vi "Synchronized Linked AI and AO.vi"() -> ()   [LabVIEW 2019, in "GettingStarted_5785_Host.lvlib"]
uses:
  GettingStarted_5785_Host.lvlib
  <vilib>/userDefined/High Color/nirio_resource_hc.ctl
  <instrlib>/FlexRIO/API/Host/v1/NI FlexRIO/API/Reference Clock Source.ctl
  <instrlib>/FlexRIO/API/Host/v1/NI FlexRIO/API/Configure Reference Clock.vi
  <instrlib>/FlexRIO/API/Host/v1/NI FlexRIO/API/Get Property Reference - Fpga Small.vi
  <instrlib>/FlexRIO/API/Host/v1/NI FlexRIO/API/Configure Immediate Start Trigger.vi
  <instrlib>/FlexRIO/API/Host/v1/NI FlexRIO/API/Configure Digital Edge Start Trigger.vi
  <instrlib>/FlexRIO/API/Host/v1/NI FlexRIO/API/Read Stream 1D WDT.vi
  <vilib>/FPGAPlugInAG/Dynamic/niLvFpga_Close_Dynamic.vi
  <vilib>/rvi/interface/nirviCloseFPGA/nirviCloseFPGA.xnode
  <instrlib>/FlexRIO/API/Host/v1/NI FlexRIO API v1.lvlib
  <resource>/objmgr/niflexrioapiStream.rc
  <resource>/objmgr/niflexrioapiTrigger.rc
panel:
  in  "flexrio tranceivers":T2(array[cluster])
  in  "frequency":dbl=32000000.0 format="%0.2p"
  in  "amplitude":dbl=0.2 format="%#_13p"
  in  "sampling info":cluster{"Fs":dbl, "#s":dbl}={"Fs"=3200000000.0, "#s"=1600.0}
  in  "samples to acquire":u64=65536
  out "error out":errorcluster
  out "read data":waveform(dbl)[](graph)=[{"t0"=timestamp(0 s since 1904-01-01), "dt"=3.125e-10, "Y"=[]}, {"t0"=timestamp(0 s since 1904-01-01), "dt"=3.125e-10, "Y"=[]}, {"t0"=timestamp(0 s since 1904-01-01), "dt"=3.125e-10, "Y"=[]}, {"t0"=timestamp(0 s since 1904-01-01), "dt"=3.125e-10, "Y"=[]}]
  out "Output Waveform":waveform(dbl)[](graph)
  in  "trigger source":string(combo)
  in  "trigger mode":enum16{"Immediate", "Digital"}(ring)
  # "This example demonstrates how to synchronize multiple FlexRIO transceivers.\nIn this example, the AO stream is linked to the AI stream, meaning that AO generation will begin after AI acquisition.\n\nFor demonstration, it's suggested to use two transceivers, with AO0 on one device connected to AI0 on the other device.\n\nThe same waveform is downloaded to each each device, and generation will begin on AO0 and AO1 when the start trigger is received. AI0 and AI1 are acquired and plotted when the start trigger is received."
  # "Acquisition trigger configuration"
  # "Digital Trigger configuration"
  # "NOTE: it is expected to see the data zeroed out at the beginning.\nThere are sampling, processing, and propagation delays in the parts, the FPGA\ninterface, etc."
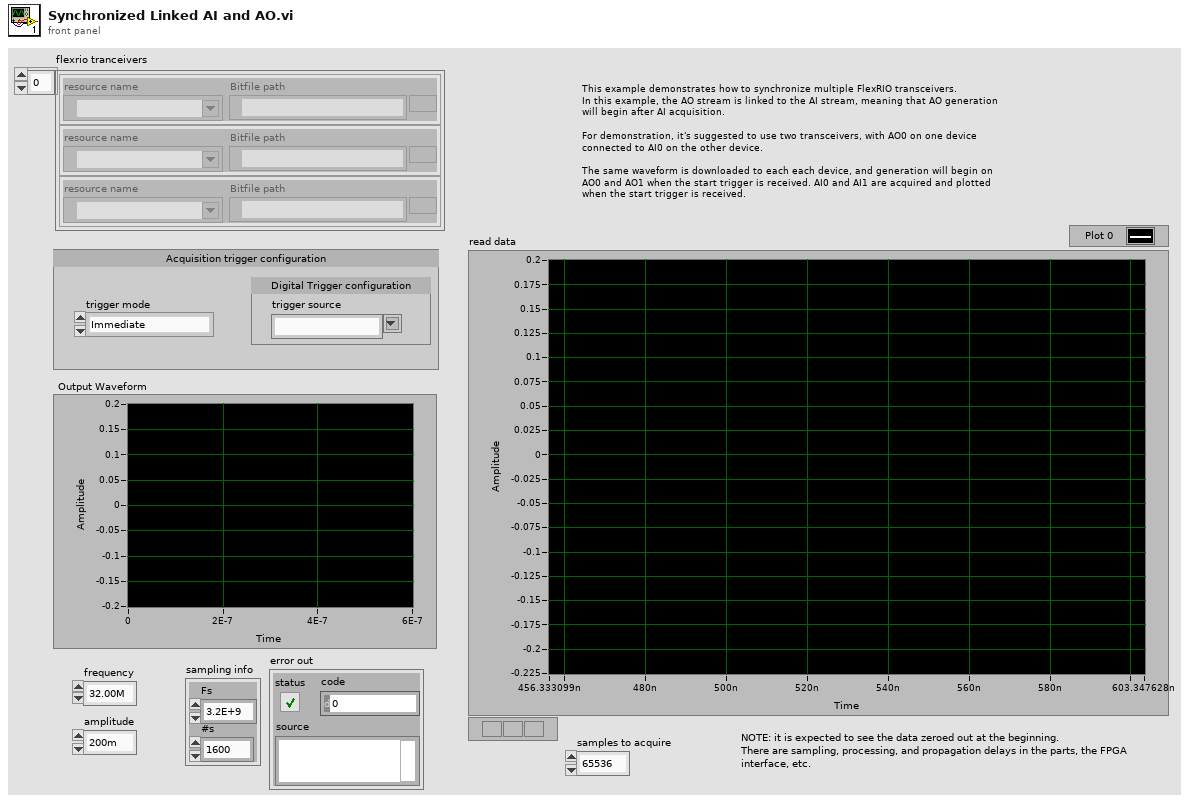
[diagram p1: front panel]
types:
  T1 = typedef "nirio_resource_hc.ctl" = tag
  T2 = cluster{"resource name":T1, "Bitfile path":path}[]
  T3 = typedef "NI FlexRIO API v1.lvlib/Reference Clock Source.ctl" = i32
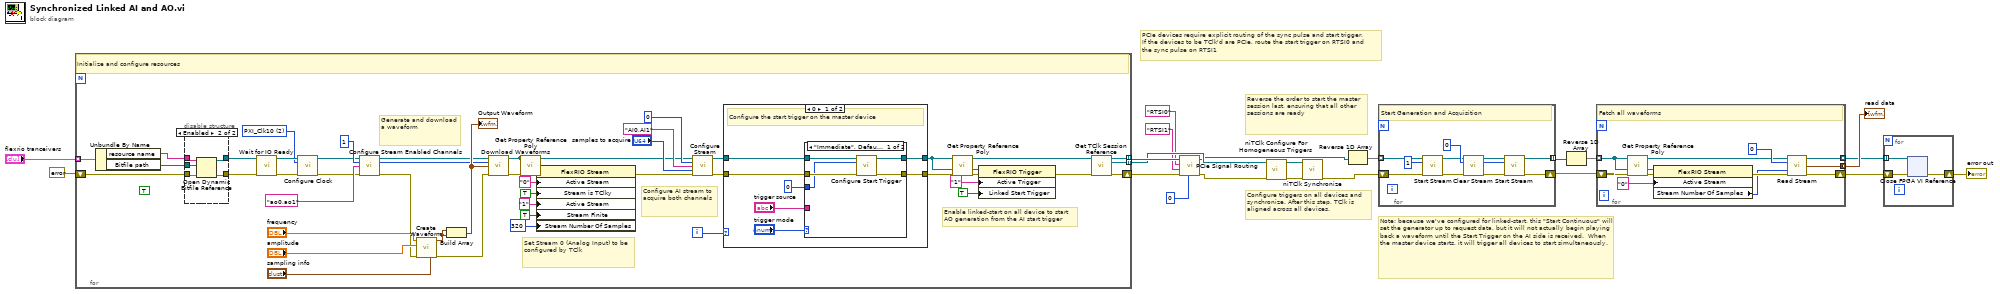
[diagram p0: block diagram]
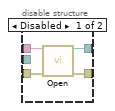
[diagram p2: hidden frame]
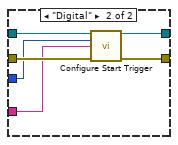
[diagram p3: hidden frame]
diagram:
  # "PCIe devices require explicit routing of the sync pulse and start trigger.\nIf the devices to be TClk'd are PCIe, route the start trigger on RTSI0 and\nthe sync pulse on RTSI1"
  # "Note: because we've configured for linked-start, this \"Start Continuous\" will set the generator up to request data, but it will not actually begin playing back a waveform until the Start Trigger on the AI side is received.  When the master device starts, it will trigger all devices to start simultaneously."
  # "Reverse the order to start the master session last, ensuring that all other sessions are ready"
  # "Configure triggers on all devices and\nsynchronize. After this step, TClk is\naligned across all devices."
  n1 = for {
    shift-right: [w49] -> w7
    shift-left: errorcluster {"status"=FALSE, "code"=0, "source"=""} ("error out") -> [w24]
    tunnel: "flexrio tranceivers" -> [w54] mode=indexing
    tunnel: [w48] -> w8 mode=indexing
    tunnel: [w47] -> w4 mode=indexing
    i -> [w50]
    w30 = T3 2 items=["Default", "Onboard", "PXI_Clk10", "External", "None", "Baseboard Reference"] ("reference clock source")
    (unwired) TRUE ("Run When Loaded")
    # "Enable linked-start on all device to start\nAO generation from the AI start trigger"
    # "Configure AI stream to acquire both channels"
    # "Set Stream 0 (Analog Input) to be configured by TClk"
    # "Generate and download a waveform"
    # "Initialize and configure resources"
    n2 = Unbundle By Name(w54) -> ("resource name"=w23:T1, "Bitfile path"=w22:path)
    n3 = disable-structure shown="Enabled" {
      disable-tunnel: [w73 w77] -> w26
      disable-tunnel: [w72 w78] -> w25
      disable-tunnel: w24 -> [w71 w74]
      disable-tunnel: w23 -> [w70 w76]
      disable-tunnel: w22 -> [_ w75]
      frame Disabled {
        n4 = call <instrlib>:"Open.vi"("RIO Device"=w70, "error in"=w71) -> ("fpga interface out"=w73:refnum<k20>, "error out"=w72:errorcluster)  [unwired: 12 in]
      }
      frame Enabled {
        n5 = Open Dynamic Bitfile Reference(0:w76, 1:w75, 3:w74) -> (5:w77:refnum<k20>, 8:w78:errorcluster)  [unwired: 2 in]
      }
    }
    n6 = call <instrlib>:"Wait for IO Ready.vi"("fpga interface in"=w26, "error in"=w25) -> ("fpga interface out"=w34:refnum<k20>, "error out"=w31:errorcluster)  [unwired: 10 in, 2 out]
    n7 = call-poly <instrlib>:"Configure Clock.vi"("fpga interface in"=w34, "reference clock source"=w30, "error in"=w31) -> ("fpga interface out"=w33:refnum<k20>, "error out"=w32:errorcluster)  [unwired: 11 in]
    n8 = call <instrlib>:"Configure Stream Enabled Channels.vi"("fpga interface in"=w33, "stream instance"=u32 1, "channels enabled"="ao0,ao1", "error in"=w32) -> ("fpga interface out"=w39:refnum<k20>, "stream instance out"=w35:u32, "error out"=w38:errorcluster)  [unwired: 8 in, 1 out]
    n9 = call "Create Waveform.vi"("sampling info"="sampling info", "error in (no error)"=w38, "amplitude"="amplitude", "frequency"="frequency") -> ("error out"=w53:errorcluster, "Output Waveform (V)"=w59:waveform(dbl))  [unwired: 5 in, 1 out]
    n10 = Build Array(w59, w59) -> (w57:waveform(dbl)[])
    "Output Waveform" <- w57
    n11 = call "Download Waveforms.vi"("fpga interface in"=w39, "stream instance"=w35, "waveforms"=w57, "error in"=w53) -> ("fpga interface out"=w58:refnum<k20>, "error out"=w56:errorcluster)  [unwired: 9 in, 1 out]
    n12 = call-poly <instrlib>:"Get Property Reference Poly.vi"("error in (no error)"=w56, "fpga interface in"=w58) -> ("error out"=w69:errorcluster, "property reference"=w68:refnum<k20>)  [unwired: 4 in, 1 out]
    n13 = property class="FlexRIO Stream"(reference=w68, error in=w69, "Active Stream"="0", "Stream is TClky"=TRUE ("Configuration:Stream is TClky"), "Active Stream"="1", "Stream Finite"=TRUE ("Configuration:Finite"), "Stream Number Of Samples"=u64 320) -> (error out=w65:errorcluster)  [unwired: 1 out]
    n14 = call <instrlib>:"Configure Stream.vi"("fpga interface in"=w58, "stream instance"=u32 0, "channels enabled"="AI0,AI1", "num samples"="samples to acquire", "error in"=w65) -> ("fpga interface out"=w52:refnum<k20>, "error out"=w51:errorcluster)  [unwired: 7 in, 2 out]
    n15 = case shown="0" w50 {
      tunnel: [w83 w98] -> w40
      tunnel: w52 -> [w82 w98]
      tunnel: w51 -> [w81 w97]
      tunnel: [w80 w97] -> w43
      frame 0 {
        # "Configure the start trigger on the master device"
        n16 = case shown="\"Immediate\", Default" "trigger mode" {
          tunnel: w81 -> [w90 w95]
          tunnel: w82 -> [w87 w96]
          tunnel: [w89 w94] -> w80
          tunnel: [w86 w93] -> w83
          tunnel: u32 0 ("trigger instance") -> [w88 w92]
          tunnel: "trigger source" -> [_ w91]
          frame "Immediate", Default {
            n17 = call-poly <instrlib>:"Configure Start Trigger.vi"("fpga interface in"=w87, "trigger instance"=w88, "error in"=w90) -> ("fpga interface out"=w86:refnum<k20>, "error out"=w89:errorcluster)  [unwired: 10 in, 1 out]
          }
          frame "Digital" {
            n18 = call-poly <instrlib>:"Configure Start Trigger.vi"("fpga interface in"=w96, "trigger instance"=w92, "trigger source"=w91, "error in"=w95) -> ("fpga interface out"=w93:refnum<k20>, "error out"=w94:errorcluster)  [unwired: 9 in, 1 out]
          }
        }
      }
      frame 1, Default {
        # "Do not configure a trigger on the slaves (TClk will)"
      }
    }
    n19 = call-poly <instrlib>:"Get Property Reference Poly.vi"("error in (no error)"=w43, "fpga interface in"=w40) -> ("error out"=w46:errorcluster, "property reference"=w45:refnum<k20>)  [unwired: 4 in, 1 out]
    n20 = property class="FlexRIO Trigger"(reference=w45, error in=w46, "Active Trigger"="1" ("Active Stream"), "Linked Start Trigger"=TRUE ("Start:Linked")) -> (error out=w41:errorcluster)  [unwired: 1 out]
    n21 = call <instrlib>:"Get TClk Session Reference.vi"("fpga interface in"=w40, "error in"=w41) -> ("fpga interface out"=w48:refnum<k20>, "tclk session reference"=w47:refnum<k20>, "error out"=w49:errorcluster)  [unwired: 11 in]
  }
  n22 = call "PCIe Signal Routing.vi"("trigger master index"=0, "error in"=w7, "sync pulse rtsi line"="RTSI1", "start trigger rtsi line"="RTSI0", "fpga interfaces in"=w8) -> ("error out"=w5:errorcluster, "fpga interfaces out"=w3:refnum<k20>[])  [unwired: 5 in]
  n23 = call <instrlib>:"niTClk Configure For Homogeneous Triggers.vi"("error in (no error)"=w5, "sessions"=w4) -> ("error out"=w21:errorcluster, "sessions out"=w20:refnum<k20>[])  [unwired: 8 in]
  n24 = call <instrlib>:"niTClk Synchronize.vi"("error in (no error)"=w21, "sessions"=w20) -> ("error out"=w18:errorcluster)  [unwired: 8 in, 1 out]
  n25 = Reverse 1D Array(array=w3) -> (reversed array=w19:refnum<k20>[])
  n26 = for {
    tunnel: w19 -> [w103] mode=indexing
    shift-right: [w109] -> w16
    shift-left: w18 -> [w102]
    tunnel: [w108] -> w17 mode=indexing
    # "Start Generation and Acquisition"
    n27 = call <instrlib>:"Start Stream.vi"("fpga interface in"=w103, "stream instance"=u32 1, "error in"=w102) -> ("fpga interface out"=w100:refnum<k20>, "error out"=w99:errorcluster)  [unwired: 10 in, 1 out]
    n28 = call <instrlib>:"Clear Stream.vi"("fpga interface in"=w100, "stream instance"=u32 0, "error in"=w99) -> ("fpga interface out"=w106:refnum<k20>, "stream instance out"=w104:u32, "error out"=w107:errorcluster)  [unwired: 10 in]
    n29 = call <instrlib>:"Start Stream.vi"("fpga interface in"=w106, "stream instance"=w104, "error in"=w107) -> ("fpga interface out"=w108:refnum<k20>, "error out"=w109:errorcluster)  [unwired: 10 in, 1 out]
  }
  n30 = Reverse 1D Array(array=w17) -> (reversed array=w15:refnum<k20>[])
  n31 = for {
    tunnel: w15 -> [w110] mode=indexing
    tunnel: [w113] -> w14 mode=concatenating
    shift-right: [w112] -> w12
    shift-left: w16 -> [w117]
    tunnel: [w111] -> w13 mode=indexing
    # "Fetch all waveforms"
    n32 = call-poly <instrlib>:"Get Property Reference Poly.vi"("error in (no error)"=w117, "fpga interface in"=w110) -> ("error out"=w120:errorcluster, "property reference"=w119:refnum<k20>)  [unwired: 4 in, 1 out]
    n33 = property class="FlexRIO Stream"(reference=w119, error in=w120, "Active Stream"="0") -> (error out=w116:errorcluster, "Stream Number Of Samples"=w115:u64)  [unwired: 1 out]
    n34 = call-poly <instrlib>:"Read Stream.vi"("fpga interface in"=w110, "stream instance"=u32 0, "samples"=w115, "error in"=w116) -> ("fpga interface out"=w111:refnum<k20>, "read data"=w113:waveform(dbl)[], "error out"=w112:errorcluster)  [unwired: 7 in, 2 out]
  }
  "read data" <- w14
  n35 = for {
    tunnel: w13 -> [w122] mode=indexing
    shift-right: [w121] -> w11
    shift-left: w12 -> [w123]
    n36 = xnode "Close FPGA VI Reference"("FPGA VI Reference In"=w122, "error in"=w123) -> ("error out"=w121:errorcluster)
  }
  "error out" <- w11
